vi "Write Motor Velocity States of Single Wheel.vi"(6 "ccw caster motor velocity states":dbl[](array[numeric]), 7 "index info":T1, 8 "error in (no error)":errorcluster, 9 "ccw motor angle states (rad)":dbl[](array[numeric]), 10 "ccw motor velocity states":dbl[](array[numeric]), 11 "steering frame in":refnum<class "NI_Robotics_Steering Frame.lvclass">) -> (0 "error out":errorcluster, 3 "steering frame out":refnum<class "NI_Robotics_Steering Frame.lvclass">)   [LabVIEW 2017, in "NI_Robotics_Steering Frame.lvclass"]
uses:
  <vilib>/robotics/Steering/Steering Frame/NI_Robotics_Steering Frame.lvclass
  <vilib>/robotics/Steering/Steering Frame/NI_Robotics_Steering Frame.lvclass/NI_Robotics_Steering Frame.ctl
  <vilib>/robotics/Steering/Wheel/Update Motor Velocity State.vi
  <vilib>/robotics/Steering/Wheel/NI_Robotics_Wheel.lvclass
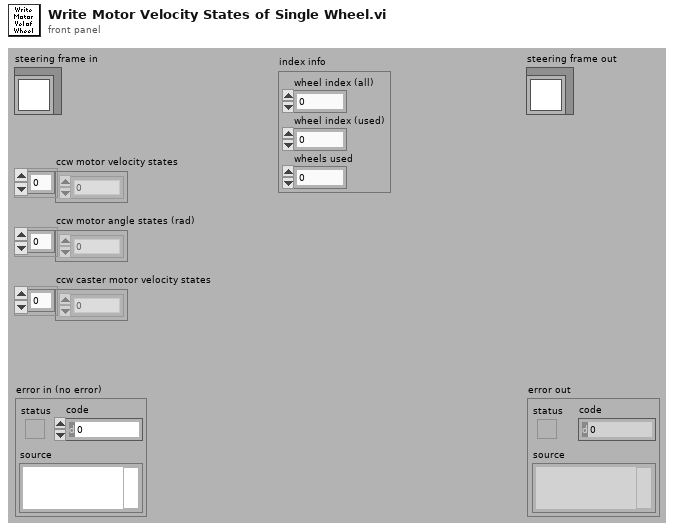
[diagram p1: front panel]
types:
  T1 = cluster{"wheel index (all)":i32, "wheel index (used)":i32, "wheels used":i32}
  T2 = typedef "NI_Robotics_Steering Frame.lvclass/Wheel Orientation.ctl" = cluster{"wheel":refnum<class "NI_Robotics_Wheel.lvclass">, "x position":dbl, "y position":dbl, "frame angle (rad)":dbl}
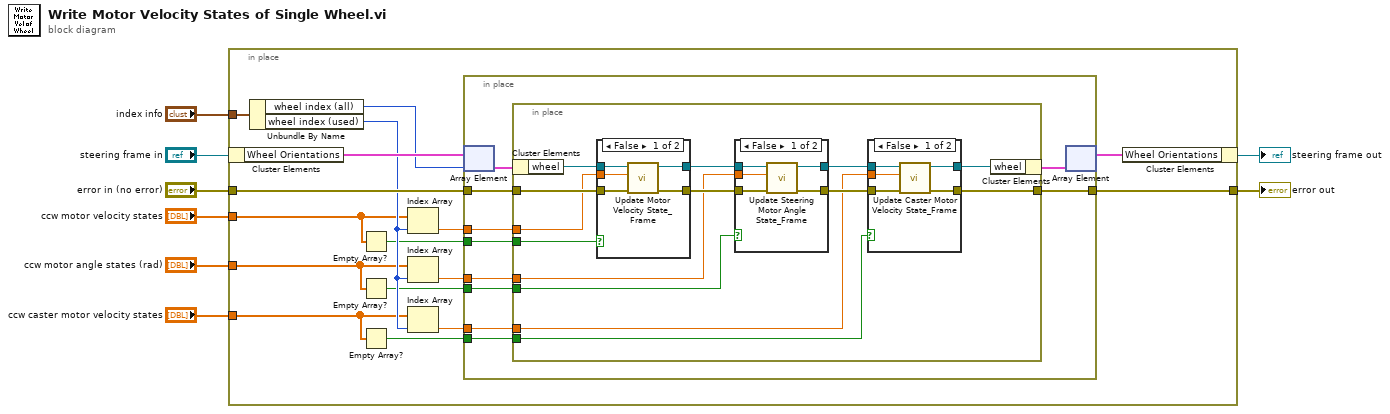
[diagram p0: block diagram]
diagram:
  n1 = in-place {
    in-place-border: "error in (no error)" -> [w24]
    in-place-border: "index info" -> [w21]
    in-place-border: "ccw caster motor velocity states" -> [w12]
    in-place-border: "ccw motor velocity states" -> [w14]
    in-place-border: "ccw motor angle states (rad)" -> [w13]
    in-place-border: [w9] -> w1
    n2 = in-place-cluster #1("steering frame in") -> ("Wheel Orientations"=w23:T2[])
    n3 = Unbundle By Name(w21) -> ("wheel index (all)"=w19:i32, "wheel index (used)"=w20:i32)
    n4 = Empty Array?(array=w14) -> (empty?=w15:bool)
    n5 = Empty Array?(array=w13) -> (empty?=w11:bool)
    n6 = Empty Array?(array=w12) -> (empty?=w10:bool)
    n7 = Index Array(array=w14, index=w20) -> (element=w18:dbl)
    n8 = Index Array(array=w13, index=w20) -> (element=w17:dbl)
    n9 = Index Array(array=w12, index=w20) -> (element=w16:dbl)
    n10 = in-place {
      in-place-border: w24 -> [w34]
      in-place-border: w18 -> [w31]
      in-place-border: w17 -> [w30]
      in-place-border: w16 -> [w29]
      in-place-border: w15 -> [w28]
      in-place-border: w11 -> [w27]
      in-place-border: w10 -> [w26]
      in-place-border: [w25] -> w9
      n11 = in-place-array #2(w23, w19) -> (w33:T2)
      n12 = in-place {
        in-place-border: w34 -> [w47]
        in-place-border: w31 -> [w46]
        in-place-border: w30 -> [w42]
        in-place-border: w29 -> [w38]
        in-place-border: w28 -> [w45]
        in-place-border: w27 -> [w41]
        in-place-border: w26 -> [w37]
        in-place-border: [w35] -> w25
        n13 = in-place-cluster #3(w33) -> ("wheel"=w48:refnum<class "NI_Robotics_Wheel.lvclass">)
        n14 = case shown="False" w45 {
          tunnel: w48 -> [w67 w68]
          tunnel: w47 -> [w66 w69]
          tunnel: w46 -> [w65 _]
          tunnel: [w64 w69] -> w43
          tunnel: [w63 w68] -> w44
          frame False {
            n15 = call <vilib>:"Update Motor Velocity State_Frame.vi"("error in (no error)"=w66, "ccw motor velocity state"=w65, "wheel in"=w67) -> ("error out"=w64:errorcluster, "wheel out"=w63:refnum<class "NI_Robotics_Wheel.lvclass">)  [unwired: 6 in, 1 out]
          }
          frame True {
          }
        }
        n16 = case shown="False" w41 {
          tunnel: w44 -> [w60 w61]
          tunnel: w43 -> [w57 w62]
          tunnel: w42 -> [w56 _]
          tunnel: [w58 w62] -> w39
          tunnel: [w59 w61] -> w40
          frame False {
            n17 = call <vilib>:"Update Steering Motor Angle State_Frame.vi"("error in (no error)"=w57, "ccw motor angle state (rad)"=w56, "wheel in"=w60) -> ("error out"=w58:errorcluster, "wheel out"=w59:refnum<class "NI_Robotics_Wheel.lvclass">)  [unwired: 6 in, 1 out]
          }
          frame True {
          }
        }
        n18 = case shown="False" w37 {
          tunnel: w40 -> [w53 w54]
          tunnel: w39 -> [w52 w55]
          tunnel: [w51 w55] -> w35
          tunnel: w38 -> [w50 _]
          tunnel: [w49 w54] -> w36
          frame False {
            n19 = call <vilib>:"Update Caster Motor Velocity State_Frame.vi"("error in (no error)"=w52, "ccw caster motor velocity state"=w50, "wheel in"=w53) -> ("error out"=w51:errorcluster, "wheel out"=w49:refnum<class "NI_Robotics_Wheel.lvclass">)  [unwired: 6 in, 1 out]
          }
          frame True {
          }
        }
        n20 = in-place-cluster #3("wheel"=w36) -> (w32:T2)
      }
      n21 = in-place-array #2(w32) -> (w22:T2[])  [unwired: 1 out]
    }
    n22 = in-place-cluster #1("Wheel Orientations"=w22) -> (→"steering frame out":refnum<class "NI_Robotics_Steering Frame.lvclass">)
  }
  "error out" <- w1
